vi "h.ACQ.GetPeaks.vi"(8 "error in":errorcluster, 10 "Timeout":i32=10000, 11 "Connection ID In":refnum<k5>) -> (0 "error out":errorcluster, 2 "Peaks Data":T1 {"Peaks Wvls, nm"."Peak Wvls, nm" format="%#_8g"}, 3 "Connection ID Out":refnum<k5>)   [LabVIEW 2019, in "h.Library.lvlib"]
doc: "This VI retrieves peaks data from a Hyperion instrument.\n\n<b>Connection ID</b> - is a network connection refnum that uniquely identifies the TCP connection\n<b>Timeout</b> - specifies the maximum amount of time, in milliseconds, for the function to complete\n<b>error in</b> - describes error conditions that occur before this node runs. This input provides standard error functionality\n<b>Connection ID out</b> - returns the same value as connection ID\n<b>Peaks Data</b> - cluster containing requested peaks wvl along with supporting data\n<b>error out</b> - contains error information. This output provides standard error out functionality."
uses:
  h.Library.lvlib
  CTL/h.ACQ.PeaksData.ctl
  CTL/h.ACQ.PeaksWvl.ctl
panel:
  # "Hyperion #GetPeaks"
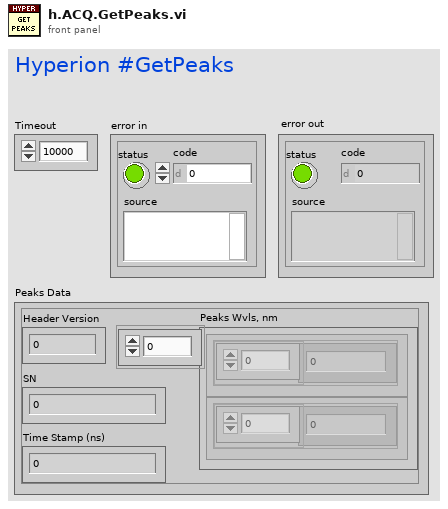
[diagram p1: front panel]
types:
  T1 = typedef "h.Library.lvlib/h.ACQ.PeaksData.ctl" = cluster{"SN":u64, "Time Stamp (ns)":u64, "Header Version":u16, "Peaks Wvls, nm":T2[]}
  T2 = typedef "h.Library.lvlib/h.ACQ.PeaksWvl.ctl" = cluster{"Peak Wvls, nm":dbl[]}
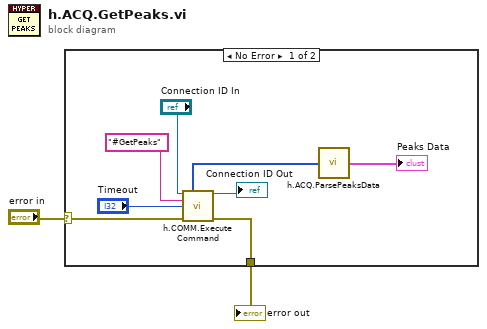
[diagram p0: block diagram]
diagram:
  n1 = case shown="No Error" "error in" {
    selector: "error in" -> [w5 w11]
    tunnel: [w4 w11] -> w1
    frame No Error {
      n2 = call "h.COMM.Execute Command.vi"("Connection ID"="Connection ID In", "Command"="#GetPeaks", "Timeout"="Timeout", "error in"=w5) -> ("Content"=w6:u8[], "Connection ID out"=→"Connection ID Out":refnum<k5>, "error out"=w4:errorcluster)  [unwired: 4 in, 5 out]
      n3 = call "h.ACQ.ParsePeaksData.vi"("Data from #GetPeaks"=w6) -> ("Peaks Data"=→"Peaks Data":T1)
    }
    frame Error {
    }
  }
  "error out" <- w1
